vi "asset.create_set_property.vi"(8 "error in":errorcluster, 9 "value":string, 10 "key":string, 11 "AssetCreateStaging in":refnum<class "AssetCreateStaging.lvclass">) -> (0 "error out":errorcluster, 3 "AssetCreateStaging out":refnum<class "AssetCreateStaging.lvclass">)   [LabVIEW 2020, in "AssetCreateStaging.lvclass"]
doc: "Sets a property key/value pair on the asset being created."
uses:
  AssetCreateStaging.lvclass
  AssetCreateStaging.lvclass/AssetCreateStaging.ctl
  client.lvlib
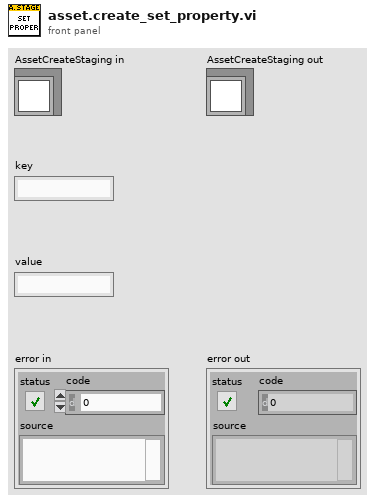
[diagram p1: front panel]
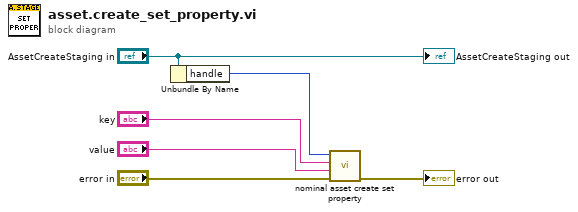
[diagram p0: block diagram]
diagram:
  n1 = Unbundle By Name("AssetCreateStaging in") -> ("handle"=w4:i32)
  n2 = call "nominal asset create set property.vi"("error in (no error)"="error in", "value"="value", "key"="key", "staging"=w4) -> ("error out"=→"error out":errorcluster)  [unwired: 6 in, 1 out]
  "AssetCreateStaging out" <- "AssetCreateStaging in"
